vi "Read Shutdown.vi"(8 "error in (no error)":errorcluster, 11 "Actor Nest in":refnum<class "Actor Nest.lvclass">) -> (0 "error out":errorcluster, 2 "Shutdown":refnum<user-event>, 3 "Actor Nest out":refnum<class "Actor Nest.lvclass">)   [LabVIEW 2012, in "Actor Nest.lvlib" / "Actor Nest.lvclass"]
uses:
  Actor Nest.lvclass
  Actor Nest.lvclass/Actor Nest.ctl
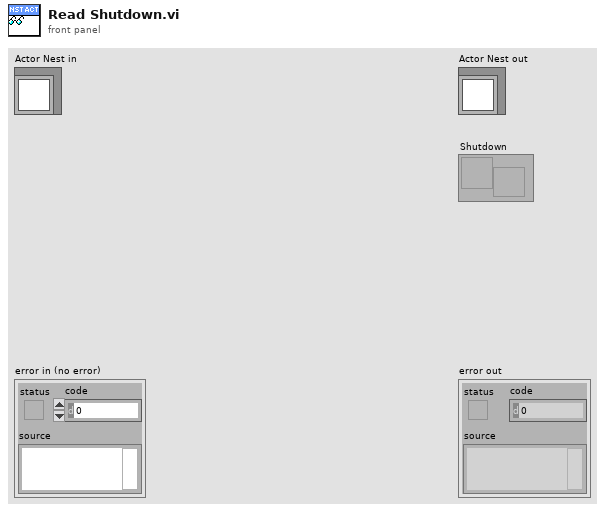
[diagram p1: front panel]
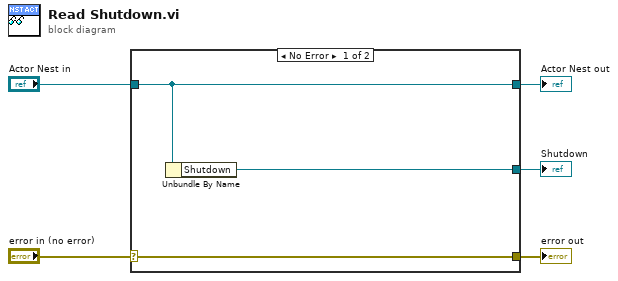
[diagram p0: block diagram]
diagram:
  n1 = case shown="No Error" "error in (no error)" {
    selector: "error in (no error)" -> [w8 w9]
    tunnel: [w8 w9] -> w4
    tunnel: [w7 w10] -> w2
    tunnel: "Actor Nest in" -> [w7 w10]
    tunnel: [w6 _] -> w1
    frame No Error {
      n2 = Unbundle By Name(w7) -> ("Shutdown"=w6:refnum<user-event>)
    }
    frame Error {
    }
  }
  "error out" <- w4
  "Actor Nest out" <- w2
  "Shutdown" <- w1
